vi "CSM - Set Log Filter Rules.vi"   [LabVIEW 2017, in "Communicable State Machine.lvlib"]
doc: "Sets global source-side filtering rules. When a log satisfies the filtering rules, the log will not be sent from the source, so no tools will be able to detect this log record.\n\n> [!NOTE]\n> This VI is a polymorphic VI. To ensure forward compatibility of the interface after modifications, it is recommended to select the instance with the newer version for this VI.\n\n\n> [!NOTE] <b>Global Log Filter Location</b>\n>\n> There are two types of global log filtering: source-side filtering and registerer-side filtering.\n>\n> - <b>Source-side filtering</b>: The CSM framework has built-in filtering rules. Based on user settings, logs can be prevented from being sent at the source.\n> - <b>Subscriber-side filtering</b>: Using the same rules, CSM provides helper VIs that can determine whether a log matches the filtering rules after it is received, allowing for different logic processing.\n>\n> Source-side processing completely prevents logs from being sent, reducing system load. Registerer-side filtering only affects the logic of that specific registerer and does not affect background log saving, offering higher flexibility.\n\n\n> [!NOTE] <b>Global Log Filter Rules</b>\n>\n> Global log filter rules allow a category of logs to be filtered out so they do not appear in the global log.\n>\n> The following are the three types of log filter rules:\n> - <b>Global Rules</b>: Apply to all modules meeting the conditions. You can configure the following settings:\n> - <b>Module Name</b>: All names of the module will be filtered.\n> - <b>Log Type</b>: Such as state, message, broadcast, module Initialization, and so on.\n> - <b>State Name</b>: Any module with the state name will be filtered.\n> - <b>State Type</b>: Type of state, such as internal state, external message, and so on.\n> - <b>Broadcast</b>: Broadcasts with the specified broadcast name will be filtered. Applies to Status Broadcast and Interrupt Broadcast logs.\n> - <b>User Log</b>: User logs with the specified user log name will be filtered.\n> - <b>Module Rules</b>: Apply to specific modules. You can configure the following settings:\n> - <b>Module Log Type</b>: Modules with the specified log types of the module are filtered.\n> - <b>State Name</b>: Modules with the specified state name are filtered.\n> - <b>State Type</b>: Modules with the specified state type are filtered.\n> - <b>Broadcast</b>: Modules with the specified broadcast name are filtered.\n> - <b>User Log</b>: Modules with the specified user log name are filtered.\n> - <b>Periodic Filter Rules</b>: This rule is currently only effective at the registration point because it is difficult to count numbers at the publication location.\n> - Whether to enable periodic filtering.\n> - <b>Threshold (#/s)</b>: Periodic filtering threshold.\n> - <b>CheckPeriod (s)</b>: Check window time.\n\n\n<b>Reference Examples</b>:\n- `4. Advance Examples\\Filter From Source(Queue).vi`\n- `4. Advance Examples\\Filter From Source(Event).vi`"
uses:
  Communicable State Machine.lvlib
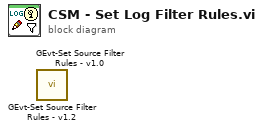
[diagram p0: block diagram]
diagram:
  n1 = call "GEvt-Set Source Filter Rules - v1.2.vi"() -> ()  [unwired: 11 in, 1 out]
  n2 = call "GEvt-Set Source Filter Rules - v1.0.vi"() -> ()  [unwired: 11 in, 1 out]
